vi "TEMOCR-Process Frame.vi"(0 "State In":T2, 2 "queue data":cluster{bool, dbl[][], "Sequence":T1}, 7 "Analysis":T3, 11 "error in (no error)":errorcluster, 13 "controls":T4) -> (4 "State Out":T2, 8 "finished":bool, 15 "error out":errorcluster)   [LabVIEW 2015]
uses:
  Typedefs/TEMOCR-Controls.ctl
  Typedefs/TEMOCR-Analysis State.ctl
  Typedefs/TEMOCR-Analysis.ctl
  Typedefs/TEMOCR-Sequence Step.ctl
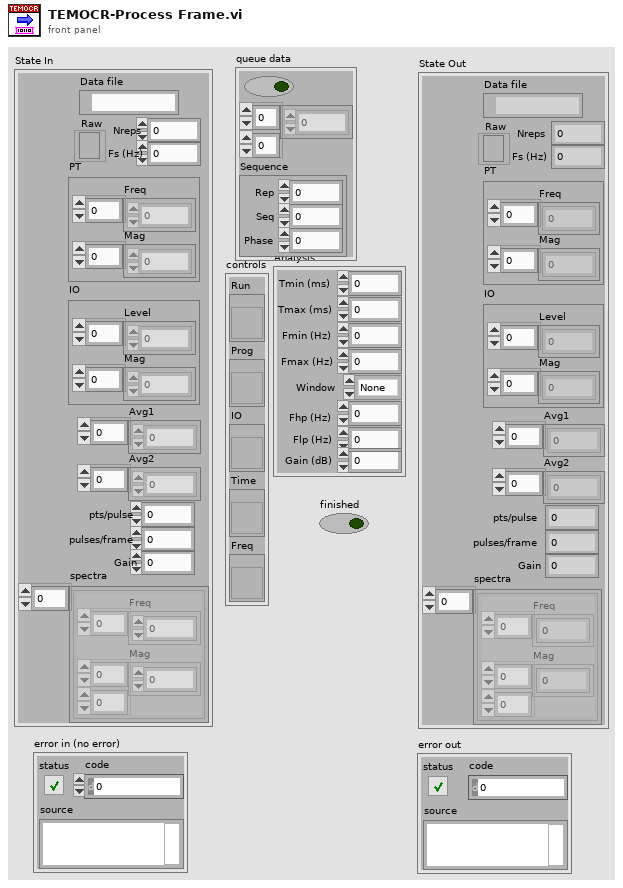
[diagram p1: front panel]
types:
  T1 = typedef "TEMOCR-Sequence Step.ctl" = cluster{"Rep":i32, "Seq":i32, "Phase":i32}
  T2 = typedef "TEMOCR-Analysis State.ctl" = cluster{"Data file":path, "Raw":refnum<file>, "PT":cluster{"Freq":dbl[], "Mag":dbl[]}, "IO":cluster{"Level":dbl[], "Mag":dbl[]}, "Nreps":i32, "Fs (Hz)":dbl, "Avg1":dbl[], "pts/pulse":i32, "pulses/frame":i32, "Avg2":dbl[], "Gain":dbl, "spectra":cluster{"Freq":dbl[], "Mag":dbl[][]}[]}
  T3 = typedef "TEMOCR-Analysis.ctl" = cluster{"Tmin (ms)":dbl, "Tmax (ms)":dbl, "Fmin (Hz)":dbl, "Fmax (Hz)":dbl, "Window":enum16{"None", "Hanning", "Hamming"}, "Fhp (Hz)":dbl, "Flp (Hz)":dbl, "Gain (dB)":dbl}
  T4 = typedef "TEMOCR-Controls.ctl" = cluster{"Run":refnum<vi>, "Prog":refnum<vi>, "IO":refnum<vi>, "Time":refnum<vi>, "Freq":refnum<vi>}
  T5 = cluster{"Freq (Hz)":dbl[], "+Freq. Mag of FFT (dB rms)":dbl[]}
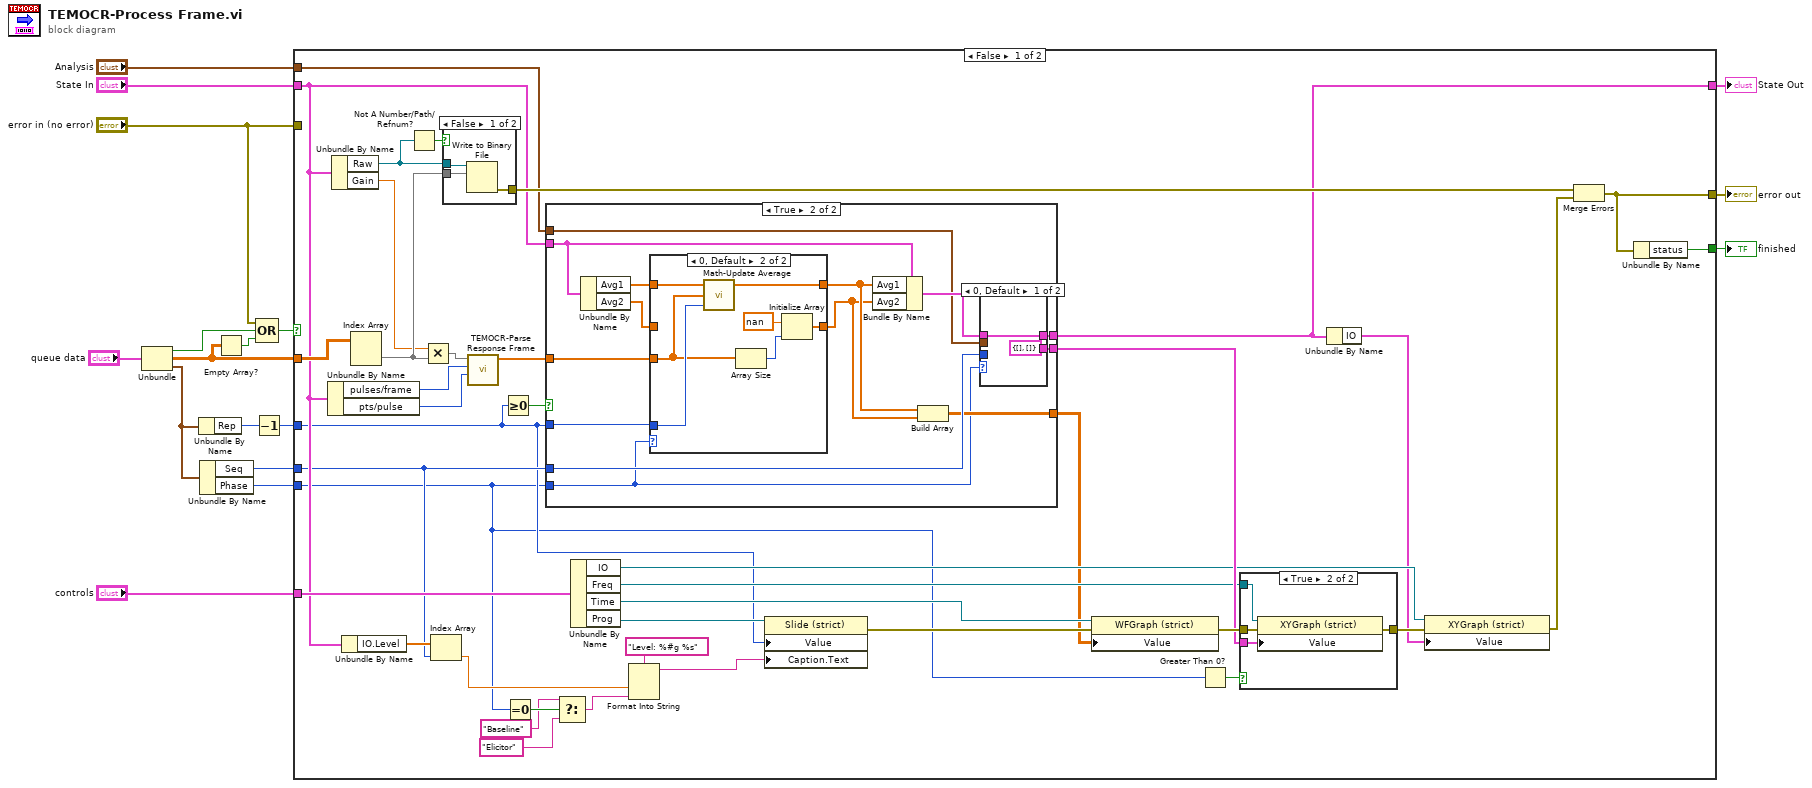
[diagram p0: block diagram]
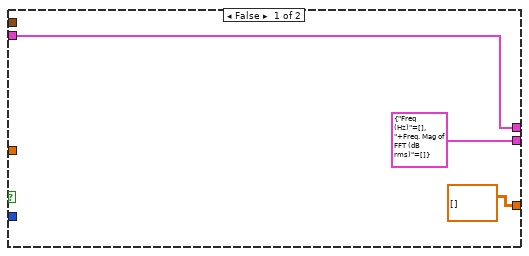
[diagram p3: hidden frame]
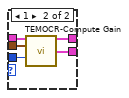
[diagram p4: hidden frame]
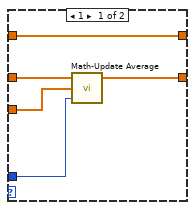
[diagram p5: hidden frame]
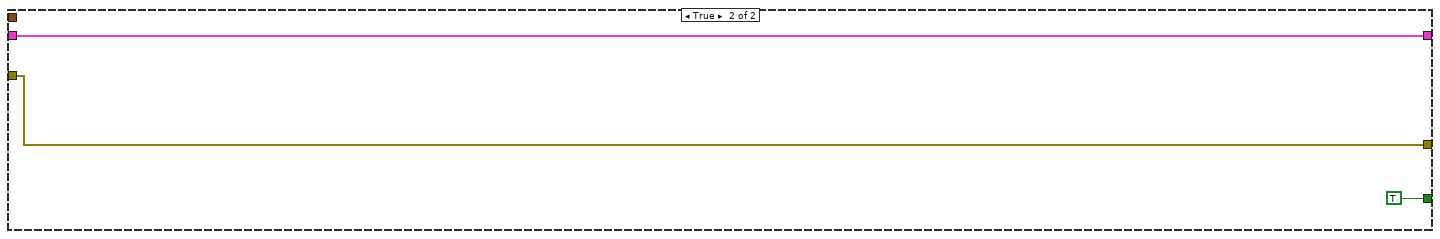
[diagram p7: hidden frame]
diagram:
  n1 = Unbundle("queue data") -> (w5:bool, w11:dbl[][], "Sequence"=w9:T1)
  n2 = Unbundle By Name(w9) -> ("Rep"=w12:i32)
  n3 = Unbundle By Name(w9) -> ("Seq"=w8:i32, "Phase"=w2:i32)
  n4 = Empty Array?(array=w11) -> (empty?=w6:bool)
  n5 = Decrement(x=w12) -> (x-1=w1:i32)
  n6 = Compound Arithmetic op=OR("error in (no error)", w5, w6) -> (w10:bool)
  n7 = case shown="False" w10 {
    tunnel: "Analysis" -> [w49 _]
    tunnel: "State In" -> [w31 w104]
    tunnel: "controls" -> [w47 _]
    tunnel: [w48 w103] -> w16
    tunnel: [w50 TRUE] -> w17
    tunnel: "error in (no error)" -> [_ w103]
    tunnel: w11 -> [w57 _]
    tunnel: w1 -> [w26 _]
    tunnel: w8 -> [w29 _]
    tunnel: [w41 w104] -> w7
    tunnel: w2 -> [w20 _]
    frame False {
      n8 = Unbundle By Name(w31) -> ("pulses/frame"=w36:i32, "pts/pulse"=w35:i32)
      n9 = Unbundle By Name(w31) -> ("Raw"=w55:refnum<file>, "Gain"=w18:dbl)
      n10 = Unbundle By Name(w31) -> ("IO.Level"=w30:dbl[])
      n11 = Index Array(array=w57) -> (element=w38:dbl[])  [unwired: 2 in]
      n12 = Not A Number/Path/Refnum?(number/path/refnum=w55) -> (NaN/Path/Refnum?=w56:bool)
      n13 = Multiply(x=w18, y=w38) -> (x*y=w19:dbl[])
      n14 = Index Array(array=w30, index=w29) -> (element=w28:dbl)
      n15 = case shown="False" w56 {
        tunnel: w55 -> [w101 _]
        tunnel: w38 -> [w100 _]
        tunnel: [w99 _] -> w51
        frame False {
          n16 = Write to Binary File(file (use dialog)=w101, data=w100) -> (error out=w99:errorcluster)  [unwired: 4 in, 2 out]
        }
        frame True {
        }
      }
      n17 = call "TEMOCR-Parse Response Frame.vi"("pts/pulse"=w35, "pulses/frame"=w36, "Array in"=w19) -> ("Array out"=w37:dbl[])  [unwired: 8 in]
      n18 = Greater Or Equal To 0?(x=w26) -> (x >= 0?=w34:bool)
      n19 = Equal To 0?(x=w20) -> (x = 0?=w25:bool)
      n20 = case shown="True" w34 {
        tunnel: w49 -> [_ w78]
        tunnel: w29 -> [_ w77]
        tunnel: [T5 {"Freq (Hz)"=[], "+Freq. Mag of FFT (dB rms)"=[]} ("freq response") w76] -> w45
        tunnel: [w65 w75] -> w41
        tunnel: w37 -> [_ w74]
        tunnel: w31 -> [w65 w72]
        tunnel: w26 -> [_ w73]
        tunnel: w20 -> [_ w66]
        tunnel: [dbl[][] [] w69] -> w33
        frame False {
        }
        frame True {
          n21 = Unbundle By Name(w72) -> ("Avg1"=w71:dbl[], "Avg2"=w70:dbl[])
          n22 = case shown="0, Default" w66 {
            tunnel: w73 -> [w88 w97]
            tunnel: w74 -> [w87 w94]
            tunnel: w71 -> [w91 w98]
            tunnel: w70 -> [w90 _]
            tunnel: [w89 w95] -> w67
            tunnel: [w91 w96] -> w68
            frame 1 {
              n23 = call "Math-Update Average.vi"("Navg In"=w88, "New sample"=w87, "Avg In"=w90) -> ("Avg Out"=w89:dbl[])  [unwired: 1 in, 1 out]
            }
            frame 0, Default {
              n24 = call "Math-Update Average.vi"("Navg In"=w97, "New sample"=w94, "Avg In"=w98) -> ("Avg Out"=w96:dbl[])  [unwired: 1 in, 1 out]
              n25 = Array Size(array=w94) -> (size(s)=w93:i32)
              n26 = Initialize Array(nan, w93) -> (w95:dbl[])
            }
          }
          n27 = Bundle By Name(cluster=w72, "Avg1"=w68, "Avg2"=w67) -> (w79:T2)
          n28 = Build Array(w68, w67) -> (w69:dbl[][])
          n29 = case shown="0, Default" w66 {
            tunnel: w79 -> [w81 w86]
            tunnel: w78 -> [_ w85]
            tunnel: w77 -> [_ w84]
            tunnel: [cluster{"Freq (Hz)":dbl[], "Mag (dB)":dbl[]} {"Freq (Hz)"=[], "Mag (dB)"=[]} ("freq response") w83] -> w76
            tunnel: [w81 w82] -> w75
            frame 0, Default {
            }
            frame 1 {
              n30 = call "TEMOCR-Compute Gain.vi"("State In"=w86, "Analysis"=w85, "seqIndex"=w84) -> ("State Out"=w82:T2, "freq response"=w83:cluster{"Freq (Hz)":dbl[], "Mag (dB)":dbl[]})  [unwired: 11 in]
            }
          }
        }
      }
      n31 = Select(t="Baseline", s=w25, f="Elicitor") -> (s? t:f=w23:string)
      n32 = Unbundle By Name(w47) -> ("IO"=w42:refnum<vi>, "Freq"=w44:refnum<vi>, "Time"=w53:refnum<vi>, "Prog"=w54:refnum<vi>)
      n33 = Format Into String(format string="Level: %#g %s", w28, w23) -> (resulting string=w27:string)  [unwired: 2 in, 1 out]
      n34 = property class="Slide (strict)"(reference=w54, "Value"=w26, "Caption.Text"=w27) -> (error out=w52:errorcluster)  [unwired: 1 in, 1 out]
      n35 = property class="WFGraph (strict)"(reference=w53, error in=w52, "Value"=w33) -> (error out=w46:errorcluster)  [unwired: 1 out]
      n36 = Greater Than 0?(x=w20) -> (x > 0?=w21:bool)
      n37 = case shown="True" w21 {
        tunnel: w46 -> [w58 w62]
        tunnel: w45 -> [_ w61]
        tunnel: w44 -> [_ w60]
        tunnel: [w58 w59] -> w43
        frame False {
        }
        frame True {
          n38 = property class="XYGraph (strict)"(reference=w60, error in=w62, "Value"=w61) -> (error out=w59:errorcluster)  [unwired: 1 out]
        }
      }
      n39 = Unbundle By Name(w41) -> ("IO"=w40:cluster{"Level":dbl[], "Mag":dbl[]})
      n40 = property class="XYGraph (strict)"(reference=w42, error in=w43, "Value"=w40) -> (error out=w39:errorcluster)  [unwired: 1 out]
      n41 = Merge Errors(w51, w39) -> (w48:errorcluster)
      n42 = Unbundle By Name(w48) -> ("status"=w50:bool)
    }
    frame True {
    }
  }
  "finished" <- w17
  "error out" <- w16
  "State Out" <- w7
